vi "ma_sml_M-1 Decimator with IC (complex input) (No State).vi"(6 "reset?":bool, 7 "sml_M-1 Decimator with IC (complex input) state in":T1={"coefficients in reverse order state"=[], "max index for coefficients state"=1} {"coefficients in reverse order state" format="%.2f"}, 8 "initial conditions":cdb[](array[numeric]) format="%.2f", 9 "M":i32=1, 10 "coefficients":dbl[](array[numeric]) format="%.2f", 11 "x":cdb[](array[numeric]) format="%.2f") -> (3 "y":cdb[](array[numeric]) format="%.2f", 4 "final conditions":cdb[](array[numeric]) format="%.2f", 5 "sml_M-1 Decimator with IC (complex input) state out":T1={"coefficients in reverse order state"=[], "max index for coefficients state"=1} {"coefficients in reverse order state" format="%.2f"})   [LabVIEW 2020, in "NI_MAPro.lvlib"]
doc: "Clockwise commutator implementation of polyphase M-1 decimator.\ncoefficients and initial conditions are in polyphase forms for the reason of computation efficiency.\nSince it is clockwise commutator model, output is one sample delayed at the output sample rate. the coefficients arrays are in the reverse order of ordinary polyphase filters."
uses:
  NI_MAPro.lvlib
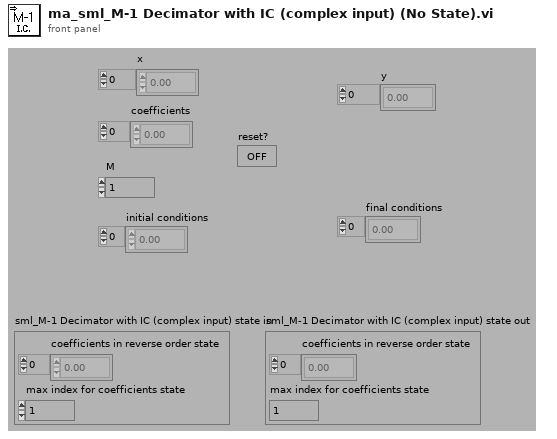
[diagram p1: front panel]
types:
  T1 = cluster{"coefficients in reverse order state":dbl[], "max index for coefficients state":i32}
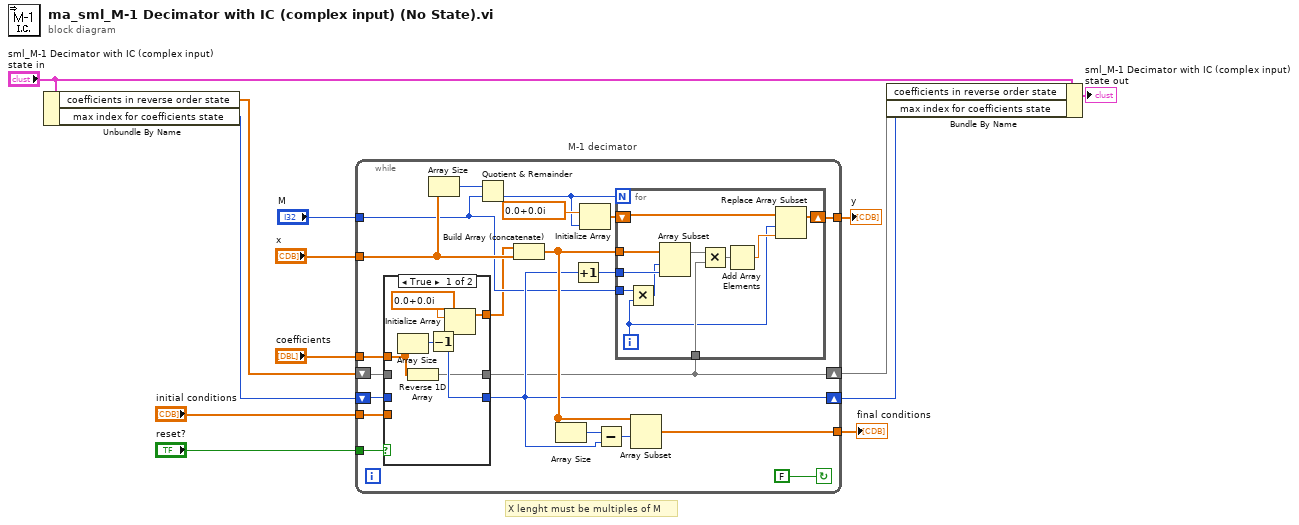
[diagram p0: block diagram]
diagram:
  # "X lenght must be multiples of M"
  # "M-1 decimator"
  n1 = Unbundle By Name("sml_M-1 Decimator with IC (complex input) state in") -> ("coefficients in reverse order state"=w6:dbl[], "max index for coefficients state"=w5:i32)
  n2 = while {
    tunnel: "M" -> [w17]
    tunnel: [w20] -> w8
    tunnel: [w24] -> w9
    tunnel: "coefficients" -> [w30]
    shift-left: w5 -> [w29]
    shift-right: [w19] -> w1
    shift-left: w6 -> [w28]
    shift-right: [w16] -> w2
    tunnel: "x" -> [w31]
    tunnel: "reset?" -> [w33]
    tunnel: "initial conditions" -> [w34]
    stop <- FALSE continue-if-true
    n3 = case shown="True" w33 {
      tunnel: w34 -> [_ w53]
      tunnel: [w46 w53] -> w15
      tunnel: w30 -> [w48 _]
      tunnel: [w49 w54] -> w19
      tunnel: w29 -> [_ w54]
      tunnel: [w47 w52] -> w16
      tunnel: w28 -> [_ w52]
      frame True {
        n4 = Array Size(array=w48) -> (size(s)=w50:i32)
        n5 = Reverse 1D Array(array=w48) -> (reversed array=w47:dbl[])
        n6 = Decrement(x=w50) -> (x-1=w49:i32)
        n7 = Initialize Array(cdb 0.0+0.0i ("Element Data"), w49) -> (w46:cdb[])
      }
      frame False {
      }
    }
    n8 = Array Size(array=w31) -> (size(s)=w32:i32)
    n9 = Quotient & Remainder(x=w32, y=w17) -> (floor(x/y)=w22:i32)  [unwired: 1 out]
    n10 = Build Array (concatenate)(w15, w31) -> (w27:cdb[])
    n11 = Array Size(array=w27) -> (size(s)=w26:i32)
    n12 = Increment(x=w19) -> (x+1=w18:i32)
    n13 = Initialize Array(cdb 0.0+0.0i ("Element Data"), w22) -> (w21:cdb[])
    n14 = Subtract(x=w26, y=w19) -> (x-y=w25:i32)
    n15 = for {
      N: w22 -> [_]
      tunnel: w27 -> [w44]
      shift-right: [w35] -> w20
      shift-left: w21 -> [w45]
      tunnel: w18 -> [w43]
      tunnel: w17 -> [w42]
      tunnel: w16 -> [w39]
      i -> [w36]
      n16 = Multiply(x=w42, y=w36) -> (x*y=w41:i32)
      n17 = Array Subset(array=w44, index=w41, length=w43) -> (w40:cdb[])
      n18 = Multiply(x=w40, y=w39) -> (x*y=w38:cdb[])
      n19 = Add Array Elements(numeric array=w38) -> (sum=w37:cdb)
      n20 = Replace Array Subset(array=w45, new element=w37, index=w36) -> (w35:cdb[])
    }
    n21 = Array Subset(array=w27, index=w25) -> (w24:cdb[])  [unwired: 1 in]
  }
  "y" <- w8
  "final conditions" <- w9
  n22 = Bundle By Name(cluster="sml_M-1 Decimator with IC (complex input) state in", "coefficients in reverse order state"=w2, "max index for coefficients state"=w1) -> (→"sml_M-1 Decimator with IC (complex input) state out":T1)
